vi "addPageBreak.vi"(8 "error in (no error)":errorcluster, 11 "WPFRun in":refnum<k24>) -> (0 "error out":errorcluster, 3 "WPFRun out":refnum<k24>)   [LabVIEW 2017, in "LabVIEW NPOI.lvlib" / "xwpfWriter.lvclass"]
uses:
  xwpfWriter.lvclass
  C:/Users/Neo/Desktop/Dev_Tools_BR/LabVIEW_NPOI/lib/NPOI 2.1.1/NPOI.OOXML.dll
  lib/NPOI 2.1.1/NPOI.OOXML.dll
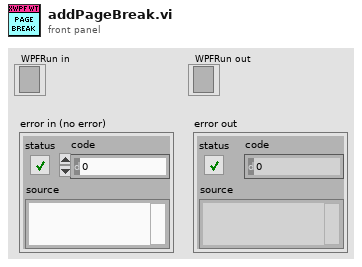
[diagram p1: front panel]
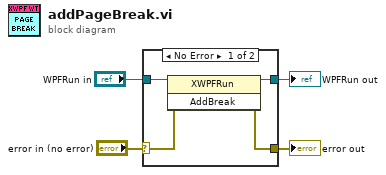
[diagram p0: block diagram]
diagram:
  n1 = case shown="No Error" "error in (no error)" {
    selector: "error in (no error)" -> [w7 w10]
    tunnel: "WPFRun in" -> [w8 w9]
    tunnel: [w6 w9] -> w2
    tunnel: [w5 w10] -> w1
    frame No Error {
      n2 = invoke class="XWPFRun" method="AddBreak"(reference=w8, error in=w7) -> (reference out=w6:refnum<k24>, error out=w5:errorcluster)  [unwired: 1 in, 1 out]
    }
    frame Error {
    }
  }
  "WPFRun out" <- w2
  "error out" <- w1
